vi "USB Multiplexor Controller.vi"(10 "Pixel number on\nsample holder":u32 caption="Pixel number on sample holder", 11 "Sample holder number":i64) -> ()   [LabVIEW 2011]
uses:
  <vilib>/ULx/Create Channel.llb/ULx Create Channel (DO-Digital Output).vi
  <vilib>/ULx/Write.llb/ULx Write (Digital U32 1Chan 1Samp).vi
panel:
  in  "Port":refnum<k21>="Dev0/AuxPort"
  in  "stop":bool
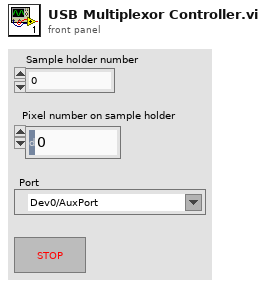
[diagram p1: front panel]
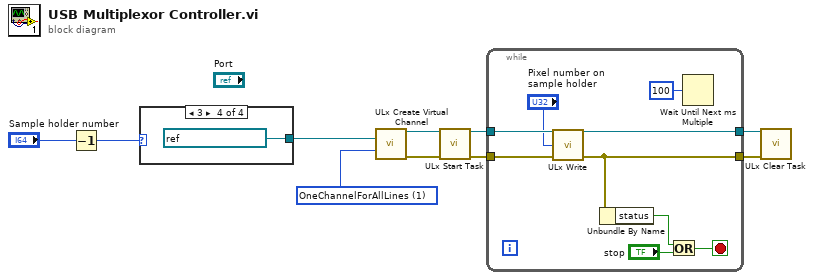
[diagram p0: block diagram]
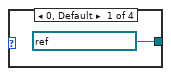
[diagram p2: hidden frame]
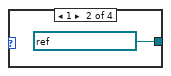
[diagram p3: hidden frame]
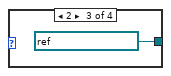
[diagram p4: hidden frame]
diagram:
  w4 = 1 items=["OneChannelForEachLine", "OneChannelForAllLines"] ("line grouping")
  n1 = Decrement(x="Sample holder number") -> (x-1=w2:i64)
  n2 = case shown="3" w2 {
    tunnel: [refnum<k21> "Dev0/1stPortA" ("Port 2") refnum<k21> "Dev0/1stPortB" ("Port 2") refnum<k21> "Dev0/1stPortA" ("Port 2") refnum<k21> "Dev0/1stPortB" ("Port 2")] -> w1
    frame 0, Default {
    }
    frame 1 {
    }
    frame 2 {
    }
    frame 3 {
    }
  }
  n3 = call-poly <vilib>:"ULx Create Virtual Channel.vi"("lines"=w1, "line grouping"=w4) -> ("task out"=w6:refnum<k24>, "error out"=w5:errorcluster)  [unwired: 12 in]
  n4 = call <vilib>:"ULx Start Task.vi"("task in"=w6, "error in"=w5) -> ("task out"=w8:refnum<k24>, "error out"=w10:errorcluster)  [unwired: 12 in]
  n5 = while {
    tunnel: w10 -> [w23]
    tunnel: [w19] -> w9
    tunnel: w8 -> [w18]
    tunnel: [w17] -> w7
    stop <- w22 stop-if-true
    n6 = call-poly <vilib>:"ULx Write.vi"("task in"=w18, "data"="Pixel number on\nsample holder", "error in"=w23) -> ("task out"=w17:refnum<k24>, "error out"=w19:errorcluster)  [unwired: 10 in, 1 out]
    n7 = Unbundle By Name(w19) -> ("status"=w20:bool)
    n8 = Or(x=w20, y="stop") -> (x .or. y?=w22:bool)
    n9 = Wait Until Next ms Multiple(millisecond multiple=u32 100 ("milliseconds to wait")) -> ()  [unwired: 1 out]
  }
  n10 = call <vilib>:"ULx Clear Task.vi"("task in"=w7, "error in"=w9) -> ()  [unwired: 13 in, 1 out]
